vi "串口配置.vi"(9 "PORT":string="1001", 10 "IP":string="127.0.0.1", 11 "请选择串口:":refnum<visa-resource-name>) -> (0 "PORT 2":string="1001", 1 "IP 2":string="127.0.0.1", 2 "确认 2":bool, 3 "VISA资源名称 2":refnum<visa-resource-name>)   [LabVIEW 2016, in "环境动力监测库.lvlib" / "空调库.lvlib"]
panel:
  in  "取消":bool
  in  "确认":bool
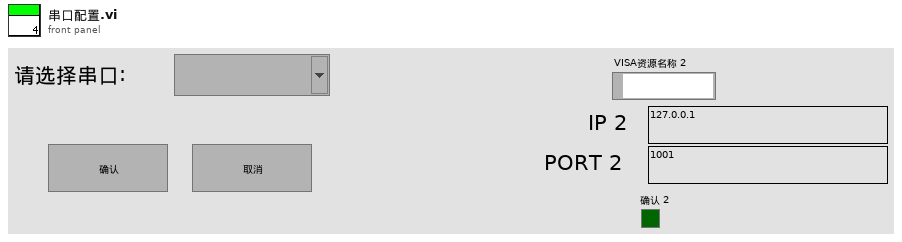
[diagram p1: front panel]
types:
  T1 = cluster{"型号选择":enum16{"黑盾", "英维克", "仁科测控RS-KTC-N01"}, "MB session in":refnum<class "MB_Master.lvclass">, "英维克空调寄存器":u16[], "通讯状态":bool, "PORT":string, "IP":string, "Slave ID ":u8, "Serial Config":cluster{"baud rate (bps)":u32, "stop bits":u16, "parity":u16, "flow control":u16, "timeout":u32, "retries":i32}, "VISA Resource":refnum<visa-resource-name>, "MB通信方式选择":enum16{"串口", "TCP"}}
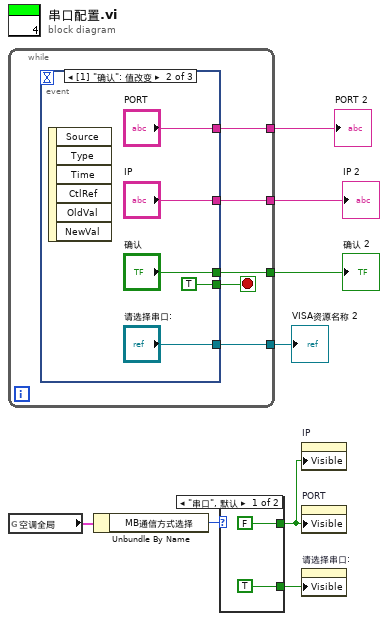
[diagram p0: block diagram]
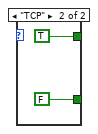
[diagram p2: hidden frame]
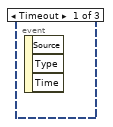
[diagram p3: hidden frame]
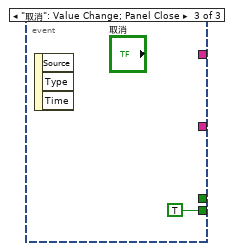
[diagram p4: hidden frame]
diagram:
  n1 = while {
    tunnel: [w13] -> w8
    tunnel: [w11] -> w7
    tunnel: [w10] -> w6
    tunnel: [w9] -> w5
    stop <- w12 stop-if-true
    n2 = event shown="[1] \"确认\": 值改变" {
      selector: _ -> [_ _ _]
      dyn-events: _ -> [_ _ _]
      timeout: _ -> [_ _ _]
      tunnel: [_ "请选择串口:" _] -> w13
      tunnel: [_ TRUE TRUE] -> w12
      tunnel: [_ "确认" _] -> w11
      tunnel: [_ "IP" _] -> w10
      tunnel: [_ "PORT" _] -> w9
      event Timeout {
        n3 = event-data() -> ()  [unwired: 1 in, 3 out]
      }
      event "确认": Value Change {
        n4 = event-data() -> ()  [unwired: 1 in, 6 out]
      }
      event "取消": Value Change; Panel Close {
        n5 = event-data() -> ()  [unwired: 1 in, 3 out]
      }
    }
  }
  "VISA资源名称 2" <- w8
  "确认 2" <- w7
  "IP 2" <- w6
  "PORT 2" <- w5
  n6 = global read "断电保存全局变量.vi" "空调全局"() -> (w2:T1)
  n7 = Unbundle By Name(w2) -> ("MB通信方式选择"=w1:enum16{"串口", "TCP"})
  n8 = case shown="\"串口\", 默认" w1 {
    tunnel: [FALSE ("可见") TRUE ("可见")] -> w4
    tunnel: [TRUE ("可见") FALSE ("可见")] -> w3
    frame "串口", Default {
    }
    frame "TCP" {
    }
  }
  n9 = property on="IP" class="Str"("Visible"=w4) -> ()  [unwired: 2 in, 2 out]
  n10 = property on="PORT" class="Str"("Visible"=w4) -> ()  [unwired: 2 in, 2 out]
  n11 = property on="请选择串口:" class="VISAName"("Visible"=w3) -> ()  [unwired: 2 in, 2 out]
